vi "ABCtoAlphaBeta_src.vi"(0 "A":sgl, 5 "B":sgl, 7 "C":sgl) -> (4 "alpha":sgl, 6 "beta":sgl)   [LabVIEW 2015]
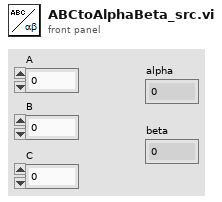
[diagram p1: front panel]
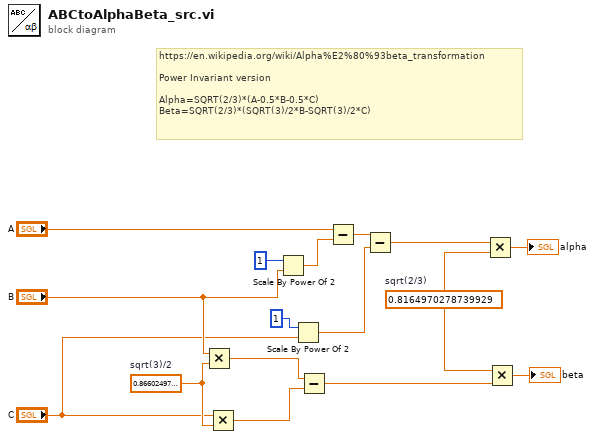
[diagram p0: block diagram]
diagram:
  w3 = sgl 0.866025  # sqrt(3)/2
  w6 = sgl 0.816497  # sqrt(2/3)
  # "https://en.wikipedia.org/wiki/Alpha%E2%80%93beta_transformation\n\nPower Invariant version\n\nAlpha=SQRT(2/3)*(A-0.5*B-0.5*C)\nBeta=SQRT(2/3)*(SQRT(3)/2*B-SQRT(3)/2*C)"
  n1 = Multiply(x="B", y=w3) -> (x*y=w4:sgl)
  n2 = Multiply(x="C", y=w3) -> (x*y=w2:sgl)
  n3 = Scale By Power Of 2(n=i16 1, x="B") -> (x*2^n=w9:sgl)
  n4 = Scale By Power Of 2(n=i16 1, x="C") -> (x*2^n=w7:sgl)
  n5 = Subtract(x=w4, y=w2) -> (x-y=w15:sgl)
  n6 = Subtract(x="A", y=w9) -> (x-y=w12:sgl)
  n7 = Subtract(x=w12, y=w7) -> (x-y=w11:sgl)
  n8 = Multiply(x=w11, y=w6) -> (x*y=→"alpha":sgl)
  n9 = Multiply(x=w6, y=w15) -> (x*y=→"beta":sgl)
